vi "ClassPanel.vi"(8 "error in (no error)":errorcluster caption="entrée d'erreur (pas d'erreur)", 11 "DK240.lvclass":refnum<class "DK240.lvclass">) -> (0 "error out":errorcluster caption="sortie d'erreur", 3 "DK240.lvclass Out":refnum<class "DK240.lvclass">)   [LabVIEW 2019, in "DK240.lvclass"]
uses:
  DK240.lvclass
  C:/Programmes Labview/LabScanV1A/DevicesClass/BaseDevice/BaseDevice.lvclass
  BaseDevice/Accessor/GetClassEvent.vi
panel:
  out "Moving":bool
  in  "Grating":u16(ring) items=["1", "2", "3"]
  in  "Lambda":dbl=60.0 caption="Position(nm)" min=-800.0 max=10000.0 step=0.01 format="%#.3f"
  in  "InSlit":u16 caption="Input Slit (mm)"
  in  "MainProgQ":refnum<queue>
  in  "MainProgQEvent":refnum<user-event>
  in  "Acq":bool
  in  "Stop":bool
  in  "MiseAJour":bool
  out "Init Program":bool
  # "DK240"
  # "this MUST labeled with class name"
  # "this MUST be present and labeled \"Stop\" and \"Acq\""
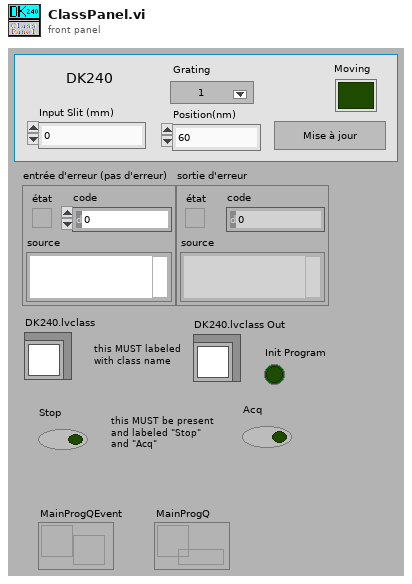
[diagram p1: front panel]
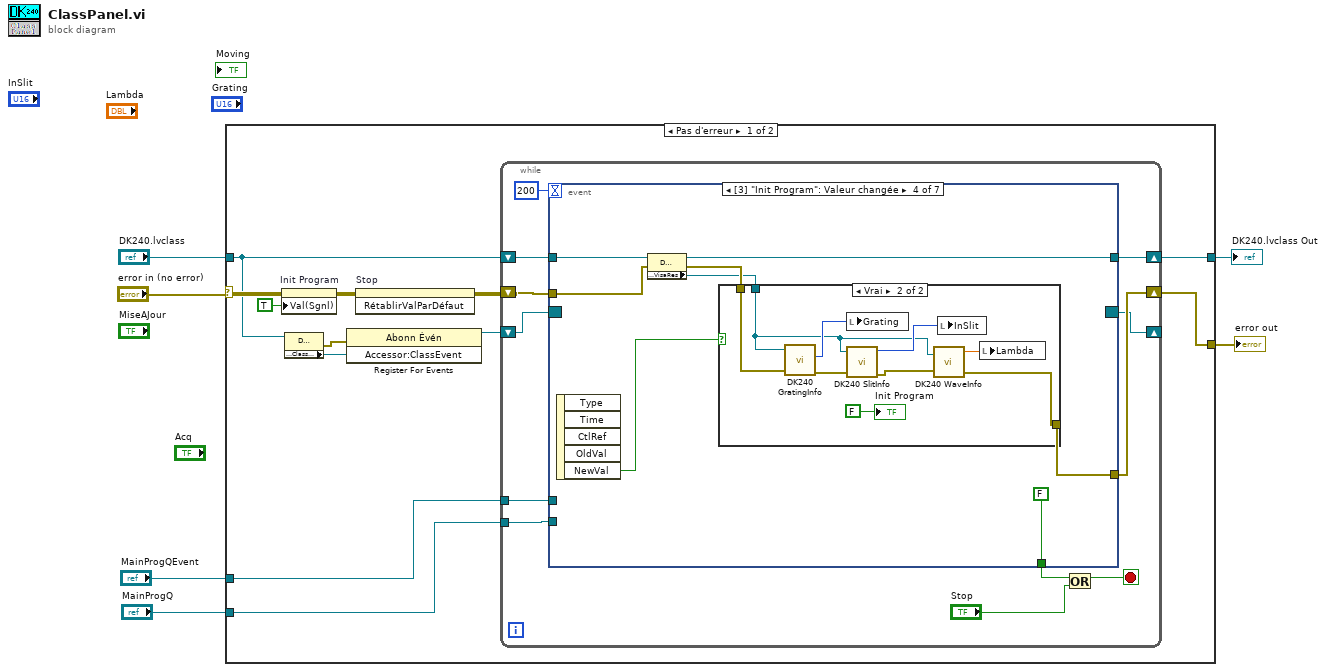
[diagram p0: block diagram]
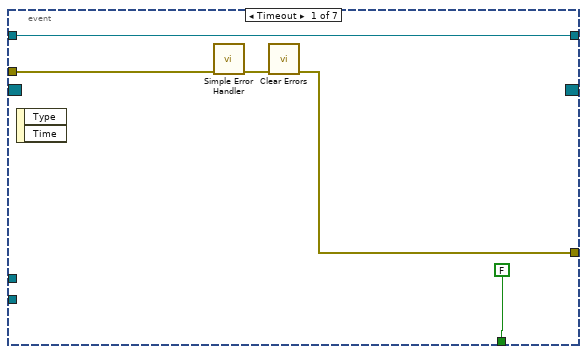
[diagram p2: hidden frame]
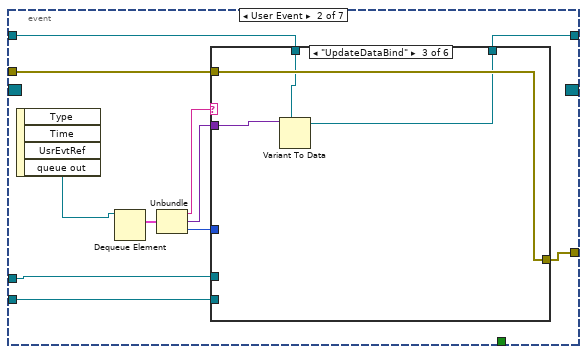
[diagram p3: hidden frame]
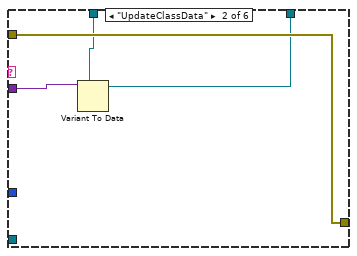
[diagram p5: hidden frame]
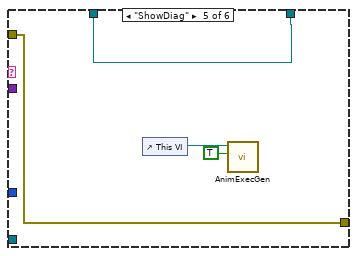
[diagram p7: hidden frame]
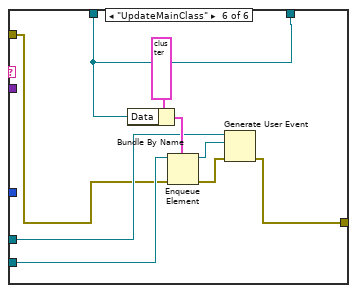
[diagram p8: hidden frame]
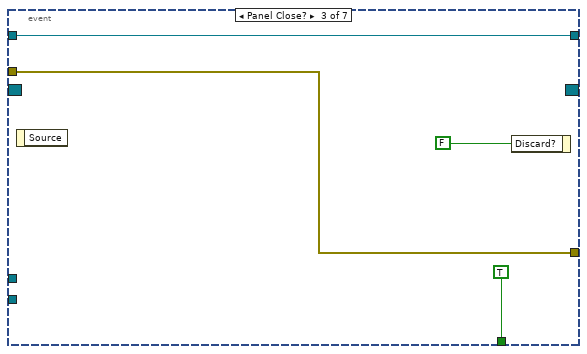
[diagram p9: hidden frame]
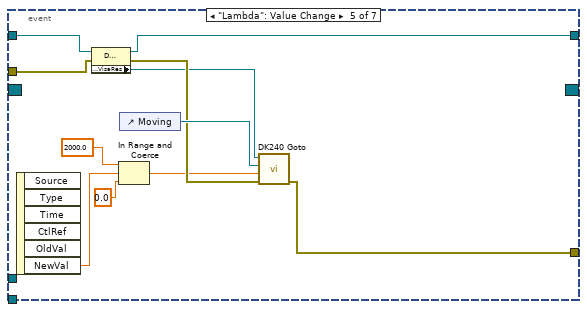
[diagram p11: hidden frame]
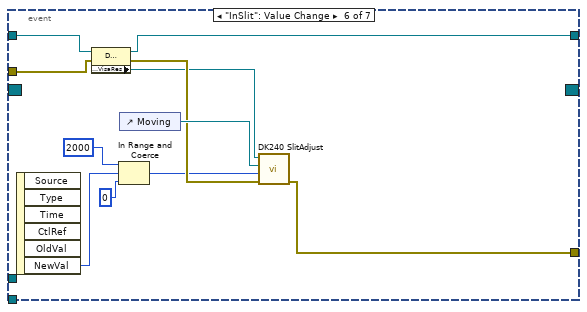
[diagram p12: hidden frame]
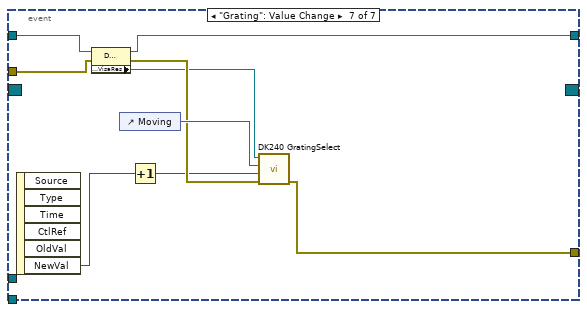
[diagram p13: hidden frame]
diagram:
  n1 = case shown="Pas d'erreur" "error in (no error)" {
    selector: "error in (no error)" -> [w15 w126]
    tunnel: [w18 w126] -> w5
    tunnel: "DK240.lvclass" -> [w10 w125]
    tunnel: [w16 w125] -> w3
    tunnel: "MainProgQEvent" -> [w8 _]
    tunnel: "MainProgQ" -> [w7 _]
    frame No Error {
      n2 = property on="Init Program" class="Bool (strict)"(error in=w15, "Val(Sgnl)"=TRUE ("Valeur (Signalisation)")) -> (error out=w14:errorcluster)  [unwired: 1 in, 1 out]
      n3 = property class="DK240.lvclass"(reference=w10) -> (error out=w12:errorcluster, "Accessor:ClassEvent"=w11:refnum<user-event>)  [unwired: 1 in, 1 out]
      n4 = register-events(error in=w12, w11) -> (reference out=w9:refnum<event-registration>)  [unwired: 1 in, 1 out]
      n5 = invoke on="Stop" class="Bool (strict)" method="RétablirValParDéfaut"(error in=w14) -> (error out=w13:errorcluster)  [unwired: 2 in, 2 out]
      n6 = while {
        shift-right: [w28] -> w18
        shift-left: w13 -> [w29]
        shift-right: [w25] -> w16
        shift-left: w10 -> [w27]
        shift-right: [w21] -> _
        shift-left: w9 -> [w22]
        tunnel: w8 -> [w20]
        tunnel: w7 -> [w19]
        stop <- w24 stop-if-true
        n7 = event shown="[3] \"Init Program\": Valeur changée" {
          selector: w22 -> [_ _ _ _ _ _ _]
          dyn-events: [_ _ _ _ _ _ _] -> w21
          timeout: 200 -> [_ _ _ _ _ _ _]
          tunnel: w29 -> [w33 w45 w73 w78 w102 w113 w122]
          tunnel: [w31 w39 w73 w82 w98 w109 w118] -> w28
          tunnel: w27 -> [w34 w46 w72 w81 w103 w114 w123]
          tunnel: [FALSE _ TRUE FALSE _ _ _] -> w26
          tunnel: [w34 w38 w72 w79 w99 w110 w119] -> w25
          tunnel: w20 -> [_ w37 _ _ _ _ _]
          tunnel: w19 -> [_ w36 _ _ _ _ _]
          event Timeout {
            n8 = event-data() -> ()  [unwired: 1 in, 2 out]
            n9 = call <vilib>:"Simple Error Handler.vi"("error in (no error)"=w33) -> ("error out"=w32:errorcluster)  [unwired: 4 in, 4 out]
            n10 = call <vilib>:"Clear Errors.vi"("error in (no error)"=w32) -> ("error out"=w31:errorcluster)  [unwired: 5 in, 1 out]
          }
          event User Event {
            n11 = event-data() -> ("queue out"=w43:refnum<queue>)  [unwired: 1 in, 3 out]
            n12 = Dequeue Element(queue=w43) -> (element=w44:cluster{"Message":string, "Data":variant, i32})  [unwired: 2 in, 3 out]
            n13 = Unbundle(w44) -> ("Message"=w42:string, "Data"=w41:variant, w40:i32)
            n14 = case shown="\"UpdateDataBind\"" w42 {
              tunnel: w45 -> [w48 w52 w56 w57 w61 w64]
              tunnel: w41 -> [_ w51 w55 _ _ _]
              tunnel: w46 -> [w47 w50 w54 w58 w62 w67]
              tunnel: [w47 w49 w53 w58 w62 w67] -> w38
              tunnel: [w48 w52 w56 w57 w61 w63] -> w39
              tunnel: w40 -> [_ _ _ _ _ _]
              tunnel: w37 -> [_ _ _ _ _ w66]
              tunnel: w36 -> [_ _ _ _ _ w65]
              frame Default {
              }
              frame "UpdateClassData" {
                n15 = Variant To Data(type=w50, Variant=w51) -> (data=w49:refnum<class "DK240.lvclass">)  [unwired: 1 in, 1 out]
              }
              frame "UpdateDataBind" {
                n16 = Variant To Data(type=w54, Variant=w55) -> (data=w53:refnum<class "DK240.lvclass">)  [unwired: 1 in, 1 out]
              }
              frame "MeasDone" {
              }
              frame "ShowDiag" {
                n17 = control-ref of="This VI"() -> (w60:refnum<vi>)
                n18 = call <userlib>:"AnimExecGen.vi"("Animer l'exécution ?"=TRUE, "ViRef"=w60) -> ()  [unwired: 9 in, 1 out]
              }
              frame "UpdateMainClass" {
                n19 = Bundle By Name(cluster=cluster{"Message":string, "Data":variant, i32} {"Message"="", "Data"=variant, 0} ("élément"), "Data"=w67) -> (w68:cluster{"Message":string, "Data":variant, i32})
                n20 = Enqueue Element(queue=w65, element=w68, error in (no error)=w64) -> (queue out=w71:refnum<queue>, error out=w70:errorcluster)  [unwired: 1 in, 1 out]
                n21 = Generate User Event(user event=w66, event data cluster=w71, error in=w70) -> (error out=w63:errorcluster)  [unwired: 1 in, 1 out]
              }
            }
          }
          event Panel Close? {
            n22 = event-data() -> ()  [unwired: 1 in, 1 out]
            n23 = event-data("Discard?"=FALSE ("Rejeter ?")) -> ()  [unwired: 1 in, 1 out]
          }
          event "Init Program": Value Change {
            n24 = event-data() -> ("NewVal"=w83:bool)  [unwired: 1 in, 4 out]
            n25 = property class="DK240.lvclass"(reference=w81, error in=w78) -> (reference out=w79:refnum<class "DK240.lvclass">, error out=w77:errorcluster, "Accessor:VisaRes"=w76:refnum<visa-resource-name>)
            n26 = case shown="Vrai" w83 {
              tunnel: w77 -> [w84 w92]
              tunnel: [w84 w86] -> w82
              tunnel: w76 -> [_ w88]
              frame False {
              }
              frame True {
                n27 = call <userlib>:"DK240 GratingInfo.vi"("error in"=w92, "Port"=w88) -> ("error out"=w90:errorcluster, "Rés act"=w91:u8)  [unwired: 1 in, 4 out]
                n28 = local write "Grating"(w91) -> ()
                n29 = call <userlib>:"DK240 SlitInfo.vi"("Port"=w88, "error in"=w90) -> ("S1 width"=w89:u16, "error out"=w87:errorcluster)  [unwired: 2 in, 2 out]
                n30 = call <userlib>:"DK240 WaveInfo.vi"("error in"=w87, "Port"=w88) -> ("error out"=w86:errorcluster, "Wavelenght"=w85:dbl)  [unwired: 2 in, 1 out]
                n31 = local write "InSlit"(w89) -> ()
                n32 = local write "Lambda"(w85) -> ()
                "Init Program" <- FALSE
              }
            }
          }
          event "Lambda": Value Change {
            n33 = event-data() -> ("NewVal"=w97:dbl)  [unwired: 1 in, 5 out]
            n34 = property class="DK240.lvclass"(reference=w103, error in=w102) -> (reference out=w99:refnum<class "DK240.lvclass">, error out=w101:errorcluster, "Accessor:VisaRes"=w100:refnum<visa-resource-name>)
            n35 = In Range and Coerce(upper limit=2000.0 ("limite supérieure"), x=w97, lower limit=0.0 ("limite inférieure")) -> (coerced(x)=w96:dbl)  [unwired: 1 out]
            n36 = control-ref of="Moving"() -> (w104:refnum<vi>)
            n37 = call <userlib>:"DK240 Goto.vi"("error in"=w101, "Wavelenght"=w96, "MovingRef"=w104, "Port"=w100) -> ("error out"=w98:errorcluster)  [unwired: 2 in, 2 out]
          }
          event "InSlit": Value Change {
            n38 = event-data() -> ("NewVal"=w108:u16)  [unwired: 1 in, 5 out]
            n39 = property class="DK240.lvclass"(reference=w114, error in=w113) -> (reference out=w110:refnum<class "DK240.lvclass">, error out=w112:errorcluster, "Accessor:VisaRes"=w111:refnum<visa-resource-name>)
            n40 = In Range and Coerce(upper limit=u16 2000 ("limite supérieure"), x=w108, lower limit=u16 0 ("limite inférieure")) -> (coerced(x)=w107:u16)  [unwired: 1 out]
            n41 = control-ref of="Moving"() -> (w115:refnum<vi>)
            n42 = call <userlib>:"DK240 SlitAdjust.vi"("error in"=w112, "SlitWidth"=w107, "MovingRef"=w115, "Port"=w111) -> ("error out"=w109:errorcluster)  [unwired: 2 in, 2 out]
          }
          event "Grating": Value Change {
            n43 = event-data() -> ("NewVal"=w117:u16)  [unwired: 1 in, 5 out]
            n44 = property class="DK240.lvclass"(reference=w123, error in=w122) -> (reference out=w119:refnum<class "DK240.lvclass">, error out=w121:errorcluster, "Accessor:VisaRes"=w120:refnum<visa-resource-name>)
            n45 = control-ref of="Moving"() -> (w124:refnum<vi>)
            n46 = Increment(x=w117) -> (x+1=w116:u16)
            n47 = call <userlib>:"DK240 GratingSelect.vi"("error in"=w121, "RésAct"=w116, "MovingRef"=w124, "Port"=w120) -> ("error out"=w118:errorcluster)  [unwired: 1 in, 2 out]
          }
        }
        n48 = Or(x=w26, y="Stop") -> (x .or. y?=w24:bool)
      }
    }
    frame Error {
    }
  }
  "error out" <- w5
  "DK240.lvclass Out" <- w3
